vi "Check for Ini files and create.vi"() -> ()   [LabVIEW 2023]
doc: "Check if class, property, and method files exist for current version of LabVIEW, and if not, create them. \n\nRead files into the property array action engine so data is ready for use.\n\nThis is launched asynchronously when plugin runs, so it should only happen once per LabVIEW version."
panel:
  out "output cluster":T1
  out "(Re)Building helper files":bool
  # "Checks for BundleMagic ini files, and if they don't exist, creates them"
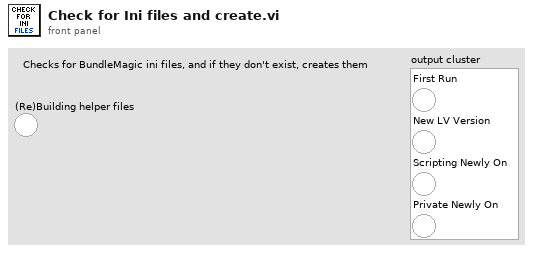
[diagram p1: front panel]
types:
  T1 = cluster{"First Run":bool, "New LV Version":bool, "Scripting Newly On":bool, "Private Newly On":bool}
  T2 = cluster{"All files found":bool, "New LV Version (no files found for current version)":bool, "First Run (no files found)":bool}
  T3 = cluster{"Class Info":cluster{"Unique ID string":string, "Parent ID string":string, "Class Name (unlocalized)":string, "Class Name (localized)":string}, "Method Info":cluster{"Unique ID string":string, "Data name":string, "Short name (localized)":string, "Long name (localized)":string}, "Method Flags":cluster{"IsDeprecated":bool, "IsPrivate":bool, "IsScripting":bool, "IsNotInRun-Time":bool}, "Divider":bool}[]
  T4 = cluster{"Class":cluster{"Unique ID string":string, "Parent ID string":string, "Class Name (unlocalized)":string, "Class Name (localized)":string}, "Property":cluster{"Unique ID string":string, "Data name":string, "Short name (localized)":string, "Long name (localized)":string}, "Flags":cluster{"CanRead":bool, "CanWrite":bool, "IsDeprecated":bool, "IsPrivate":bool, "IsScripting":bool, "IsNotInRun-Time":bool, "Is Reference":bool, "Class Name":string}, "Divider":bool, "Is Write":bool, "Unwired":bool}[]
  T5 = cluster{"Class Info":cluster{"Unique ID string":string, "Parent ID string":string, "Class Name (unlocalized)":string, "Class Name (localized)":string}, "Class Heirarchy":string, "Class Type":enum16{"Unknown", "Base", "Scripting", "Private", "Deprecated", "None", "Divider"}, "Indent":u32}[]
  T6 = cluster{"Done":refnum<user-event>, "Msg 1":refnum<user-event>, "Msg 2":refnum<user-event>, "Prog Max":refnum<user-event>, "Prog Ct":refnum<user-event>}
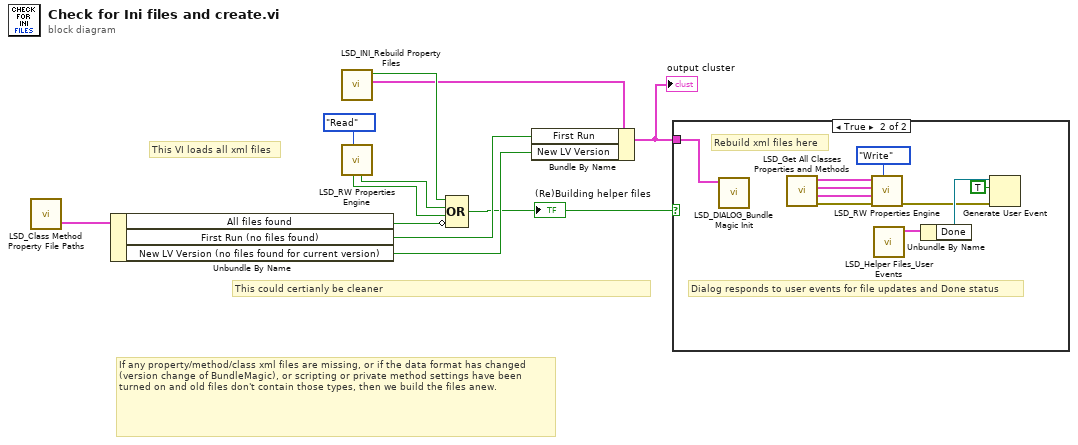
[diagram p0: block diagram]
diagram:
  # "This could certianly be cleaner"
  # "If any property/method/class xml files are missing, or if the data format has changed (version change of BundleMagic), or scripting or private method settings have been turned on and old files don't contain those types, then we build the files anew."
  # "This VI loads all xml files"
  n1 = call <resource>:"LSD_Class Method Property File Paths.vi"() -> ("Files Found Cluster"=w7:T2)  [unwired: 7 in, 4 out]
  n2 = Unbundle By Name(w7) -> ("All files found"=w6:bool, "First Run (no files found)"=w4:bool, "New LV Version (no files found for current version)"=w3:bool)
  n3 = call <resource>:"LSD_INI_Rebuild Property Files.vi"() -> ("Why are we here?"=w5:T1, "Rebuild Property Files"=w11:bool)  [unwired: 10 in]
  n4 = call <resource>:"LSD_RW Properties Engine.vi"("File Action [Read]"=enum16{"Read", "Write"}."Read") -> ("data missing?"=w8:bool, "Data format changed"=w9:bool)  [unwired: 5 in, 4 out]
  n5 = Compound Arithmetic op=OR(w11, w8, w9, invert w6) -> (w1:bool)
  "(Re)Building helper files" <- w1
  n6 = Bundle By Name(cluster=w5, "First Run"=w4, "New LV Version"=w3) -> (w2:T1)
  "output cluster" <- w2
  n7 = case shown="True" w1 {
    tunnel: w2 -> [_ w12]
    frame False {
    }
    frame True {
      # "Dialog responds to user events for file updates and Done status"
      # "Rebuild xml files here"
      n8 = call <resource>:"LSD_DIALOG_Bundle Magic Init.vi"("Why are we here?"=w12) -> ()  [unwired: 11 in]
      n9 = call <resource>:"LSD_Get All Classes Properties and Methods.vi"() -> ("error out"=w17:errorcluster, "Methods[]"=w18:T3, "Properties[]"=w19:T4, "Classes[]"=w20:T5)  [unwired: 8 in]
      n10 = call <resource>:"LSD_RW Properties Engine.vi"("File Action [Read]"=enum16{"Read", "Write"}."Write", "error in"=w17, "Methods[]"=w18, "Properties[]"=w19, "Classes[]"=w20) -> ("error out"=w13:errorcluster)  [unwired: 1 in, 5 out]
      n11 = call <resource>:"LSD_Helper Files_User Events.vi"() -> ("Init Dialog UEs"=w16:T6)  [unwired: 11 in]
      n12 = Unbundle By Name(w16) -> ("Done"=w15:refnum<user-event>)
      n13 = Generate User Event(user event=w15, event data cluster=TRUE ("event data"), error in=w13) -> ()  [unwired: 1 in, 2 out]
    }
  }
